vi "add channel to active array.vi"(2 "line to add":u32, 3 "line array in":u32[](array[numeric])) -> (0 "addition":bool, 1 "line array out":u32[](array[numeric]))   [LabVIEW 2015]
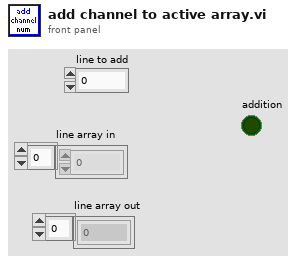
[diagram p1: front panel]
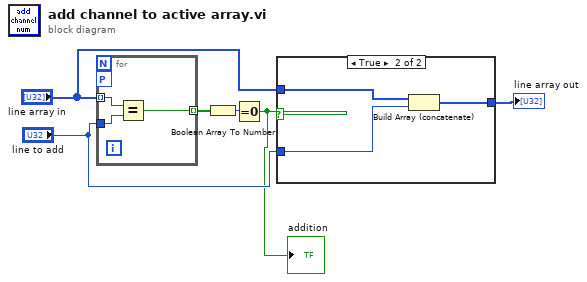
[diagram p0: block diagram]
diagram:
  n1 = for {
    workers-P: _ -> [_]
    tunnel: "line array in" -> [w8] mode=indexing
    tunnel: "line to add" -> [w9]
    tunnel: [w7] -> w6 mode=indexing
    n2 = Equal?(x=w8, y=w9) -> (x = y?=w7:bool)
  }
  n3 = Boolean Array To Number(Boolean array=w6) -> (number=w5:u32)
  n4 = Equal To 0?(x=w5) -> (x = 0?=w1:bool)
  "addition" <- w1
  n5 = case shown="True" w1 {
    tunnel: "line to add" -> [_ w12]
    tunnel: "line array in" -> [w10 w13]
    tunnel: [w10 w11] -> w2
    frame False {
    }
    frame True {
      n6 = Build Array (concatenate)(w13, w12) -> (w11:u32[])
    }
  }
  "line array out" <- w2
